vi "PathPlanner_GridPosition_FromHash.vi"(11 "Hash":i32) -> (3 "GridPosition":T1)   [LabVIEW 2019, in "PathPlanner24.lvlib"]
uses:
  PathPlanner24.lvlib
  TypeDef/PathPlannerFinderGridPosition.ctl
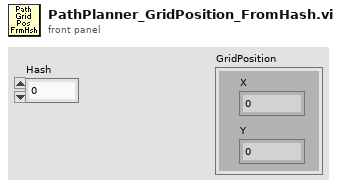
[diagram p1: front panel]
types:
  T1 = typedef "PathPlanner24.lvlib/PathPlannerFinderGridPosition.ctl" = cluster{"X":i32, "Y":i32}
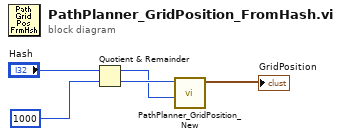
[diagram p0: block diagram]
diagram:
  n1 = Quotient & Remainder(x="Hash", y=1000) -> (x-y*floor(x/y)=w1:i32, floor(x/y)=w2:i32)
  n2 = call "PathPlanner_GridPosition_New.vi"("Int Y"=w1, "Int X"=w2) -> ("GridPosition"=→"GridPosition":T1)  [unwired: 9 in]
